vi "Enqueue.vi"(7 "Method (Back)":enum8{"Back", "Front", "Lossy", "Absent"}(ring), 8 "error in (no error)":errorcluster, 10 "Element":string, 11 "Queue in":refnum<queue>) -> (0 "error out":errorcluster, 3 "Queue out":refnum<queue>)   [LabVIEW 2018, in "QueueTimer.lvlib"]
doc: "Enqueue <b>Element</b> to <b>Queue</b>.\n\n| Method | Description |\n| --- | --- |\n| Back | Enqueue to back (last out) |\n| Front | Enqueue to front (first out) |\n| Lossy | Enqueue to back, drop front if queue is full |\n| Absent | Enqueue to back only if the element does not exist on the queue (Default) |"
uses:
  QueueTimer.lvlib
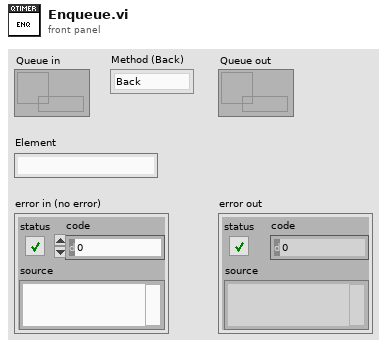
[diagram p1: front panel]
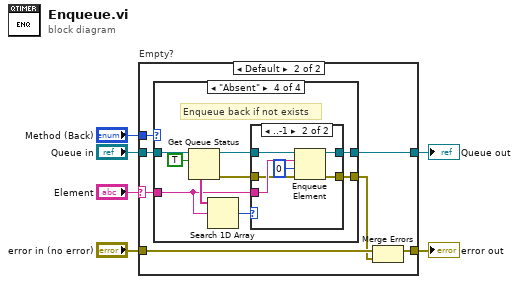
[diagram p0: block diagram]
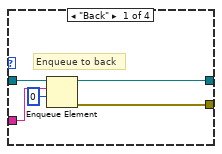
[diagram p3: hidden frame]
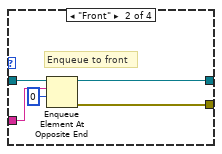
[diagram p4: hidden frame]
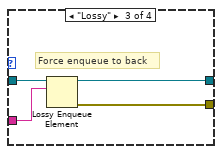
[diagram p5: hidden frame]
diagram:
  n1 = case "Empty?" shown="Default" "Element" {
    selector: "Element" -> [_ w9]
    tunnel: "Queue in" -> [w8 w15]
    tunnel: [w8 w14] -> w5
    tunnel: "error in (no error)" -> [w7 w13]
    tunnel: [w7 w12] -> w3
    tunnel: "Method (Back)" -> [_ w10]
    frame "" {
    }
    frame Default {
      n2 = case shown="\"Absent\"" w10 {
        tunnel: w15 -> [w20 w25 w29 w38]
        tunnel: [w19 w24 w28 w35] -> w14
        tunnel: [w18 w23 w27 w34] -> w11
        tunnel: w9 -> [w16 w21 w26 w32]
        frame "Back" {
          # "Enqueue to back"
          n3 = Enqueue Element(queue=w20, element=w16, timeout in ms (-1)=0) -> (queue out=w19:refnum<queue>, error out=w18:errorcluster)  [unwired: 1 in, 1 out]
        }
        frame "Front" {
          # "Enqueue to front"
          n4 = Enqueue Element At Opposite End(queue=w25, element=w21, timeout in ms (-1)=0) -> (queue out=w24:refnum<queue>, error out=w23:errorcluster)  [unwired: 1 in, 1 out]
        }
        frame "Lossy" {
          # "Force enqueue to back"
          n5 = Lossy Enqueue Element(queue=w29, element=w26) -> (queue out=w28:refnum<queue>, error out=w27:errorcluster)  [unwired: 1 in, 2 out]
        }
        frame "Absent" {
          # "Enqueue back if not exists"
          n6 = Get Queue Status(queue=w38, return elements? (F)=TRUE) -> (queue out=w36:refnum<queue>, error out=w30:errorcluster, elements=w33:string[])  [unwired: 1 in, 5 out]
          n7 = Search 1D Array(1D array=w33, element=w32) -> (index of element=w31:i32)  [unwired: 1 in]
          n8 = case shown="..-1" w31 {
            tunnel: w36 -> [w40 w46]
            tunnel: [w40 w45] -> w35
            tunnel: [w39 w44] -> w34
            tunnel: w32 -> [_ w43]
            tunnel: w30 -> [w39 w41]
            frame 0.. {
            }
            frame ..-1 {
              n9 = Enqueue Element(queue=w46, element=w43, timeout in ms (-1)=0, error in (no error)=w41) -> (queue out=w45:refnum<queue>, error out=w44:errorcluster)  [unwired: 1 out]
            }
          }
        }
      }
      n10 = Merge Errors(w13, w11) -> (w12:errorcluster)
    }
  }
  "error out" <- w3
  "Queue out" <- w5
